vi "Lab3_main.vi"() -> ()   [LabVIEW 2022 SP3]
panel:
  out "Position Error":dbl(graph)
  out "Simulation":T1(graph)
  in  "System Parameters":cluster{"a1":dbl, "a0":dbl, "a2 ":dbl, "b":dbl}={"a1"=0.1894, "a0"=0.0, "a2 "=0.0052, "b"=0.3334}
  in  "Ring":u16(ring) items=["square", "triangle", "sinusoidal"]
  in  "Frequency":dbl
  in  "Amplitude":dbl
  in  "dt (s)":dbl
  in  "On/Off":bool
  out "?":bool
  in  "stop":bool
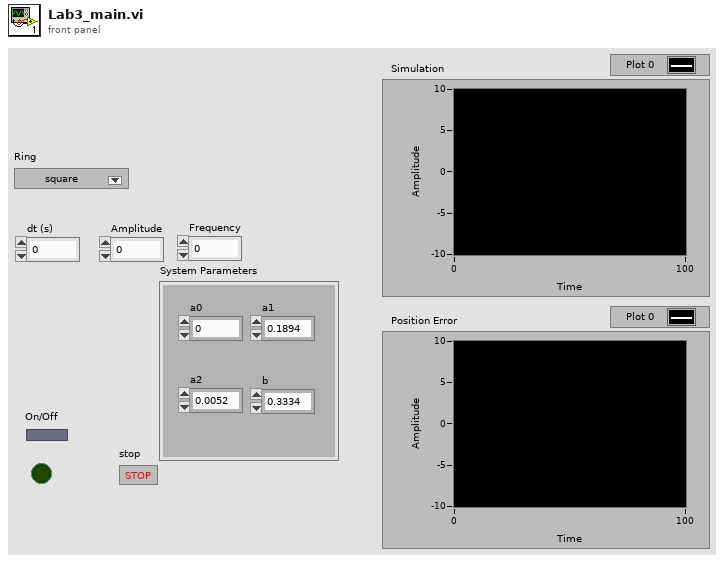
[diagram p1: front panel]
types:
  T1 = cluster{"Theta Out":dbl, "Signal Gen":dbl, "position (rad)":dbl}
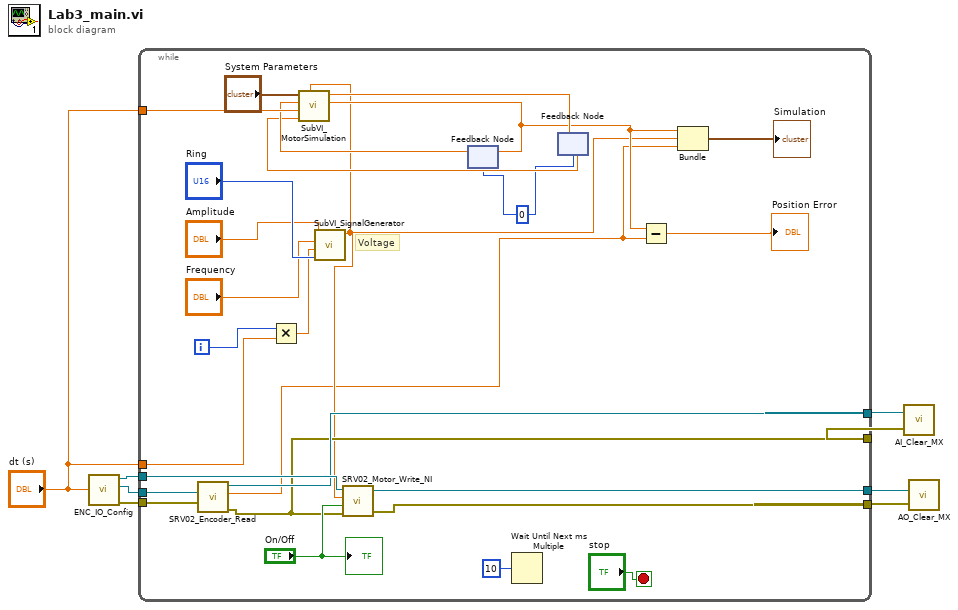
[diagram p0: block diagram]
diagram:
  n1 = call "ENC_IO_Config.vi"("dt"="dt (s)") -> ("AO Task"=w3:refnum<k21>, "ENC Task"=w4:refnum<k21>, "IO error out"=w5:errorcluster)  [unwired: 2 in, 1 out]
  n2 = while {
    tunnel: [w32] -> w8
    tunnel: [w31] -> w7
    tunnel: "dt (s)" -> [w30]
    tunnel: "dt (s)" -> [w23]
    tunnel: w5 -> [w18]
    tunnel: w4 -> [w17]
    tunnel: w3 -> [w16]
    tunnel: [w15] -> w2
    tunnel: [w14] -> w1
    i -> [w29]
    stop <- "stop" stop-if-true
    w19 = 0
    # "Voltage"
    n3 = call "SRV02_Encoder_Read.vi"("task/channels in"=w17, "error in"=w18) -> ("task out"=w15:refnum<k21>, "position (rad)"=w10:dbl, "error out"=w14:errorcluster)  [unwired: 1 out]
    n4 = Multiply(x=w29, y=w30) -> (x*y=w25:dbl)
    n5 = call "SubVI_SignalGenerator.vi"("Signal Type"="Ring", "Time"=w25, "Freq"="Frequency", "Amplitude"="Amplitude") -> ("Signal Gen"=w11:dbl)  [unwired: 7 in]
    n6 = call "SRV02_Motor_Write_NI.vi"("error in"=w14, "operate?"="On/Off", "u (V)"=w11, "task in"=w16) -> ("error out"=w31:errorcluster, "task out"=w32:refnum<k21>)  [unwired: 1 out]
    n7 = feedback #1(w19) -> (w22:dbl)
    n8 = Wait Until Next ms Multiple(millisecond multiple=10) -> ()  [unwired: 1 out]
    n9 = feedback #2(w19) -> (w20:dbl)
    n10 = call "SubVI_MotorSimulation.vi"("Input Voltage"=w11, "Velocity Reading"=w20, "dt [s]"=w23, "Position Reading"=w22, "System Parameters"="System Parameters") -> ("Theta Out"=w12:dbl, "Thetadot Out"=w21:dbl)  [unwired: 5 in]
    n11 = feedback-in #1(w12) -> ()
    n12 = feedback-in #2(w21) -> ()
    n13 = Subtract(x=w12, y=w10) -> (x-y=→"Position Error":dbl)
    n14 = Bundle("Theta Out"=w12, "Signal Gen"=w11, "position (rad)"=w10) -> (→"Simulation":T1)  [unwired: 1 in]
    "?" <- "On/Off"
  }
  n15 = call "AI_Clear_MX.vi"("Error in"=w1, "Task in"=w2) -> ()  [unwired: 1 out]
  n16 = call "AO_Clear_MX.vi"("Error in"=w7, "Task in"=w8) -> ()  [unwired: 1 out]
